vi "Update State Data.vi"(8 "error in (no error)":errorcluster, 9 "Data":variant, 10 "Argument":string, 11 "Timing Action in":refnum<class "Timing Action.lvclass">) -> (0 "error out":errorcluster, 3 "Timing Action out":refnum<class "Timing Action.lvclass">)   [LabVIEW 2020, in "MacroAssert.lvlib" / "Timing Action.lvclass"]
uses:
  Timing Action.lvclass
  Action Step/Action Step.lvclass
  Timing Action.lvclass/Timing Action.ctl
  Timing Action Type.ctl
  Time Unit.ctl
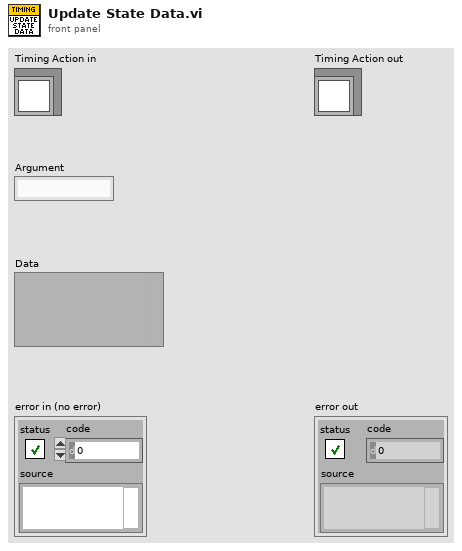
[diagram p1: front panel]
types:
  T1 = typedef "MacroAssert.lvlib/Timing Action.lvclass/Timing Action Type.ctl" = enum16{"Wait", "Wait Until"}
  T2 = typedef "MacroAssert.lvlib/Timing Action.lvclass/Time Unit.ctl" = enum16{"milliseconds", "seconds", "minutes"}
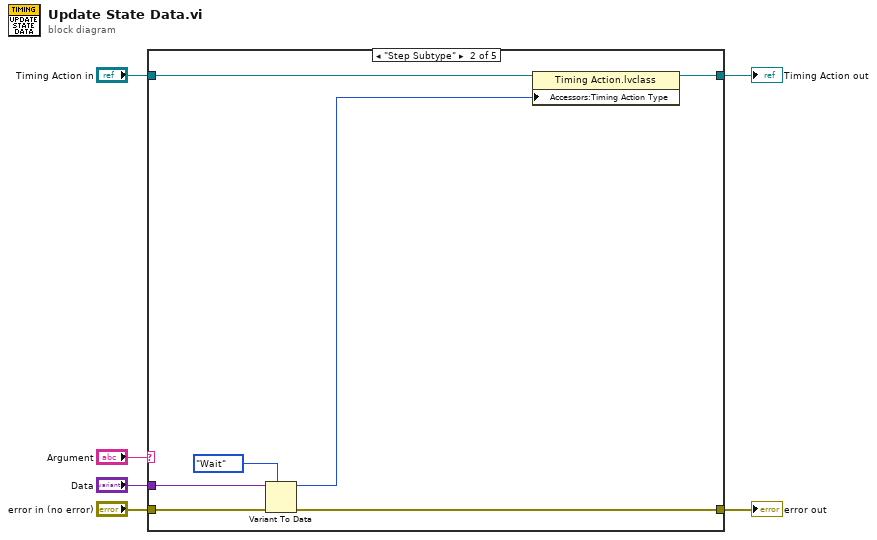
[diagram p0: block diagram]
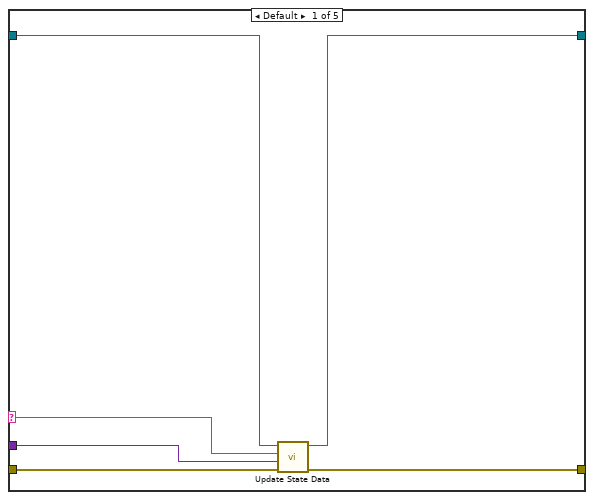
[diagram p2: hidden frame]
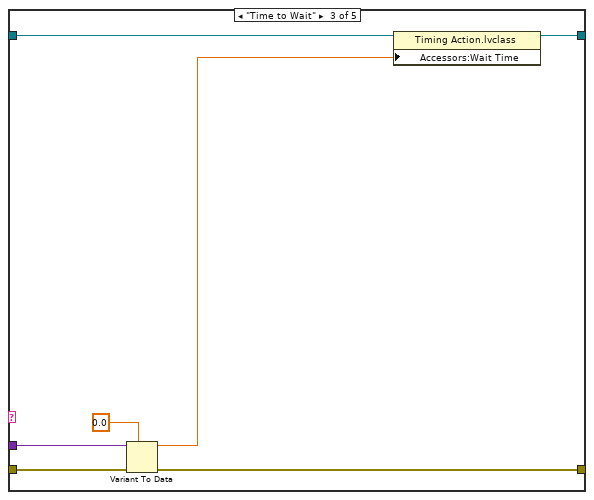
[diagram p3: hidden frame]
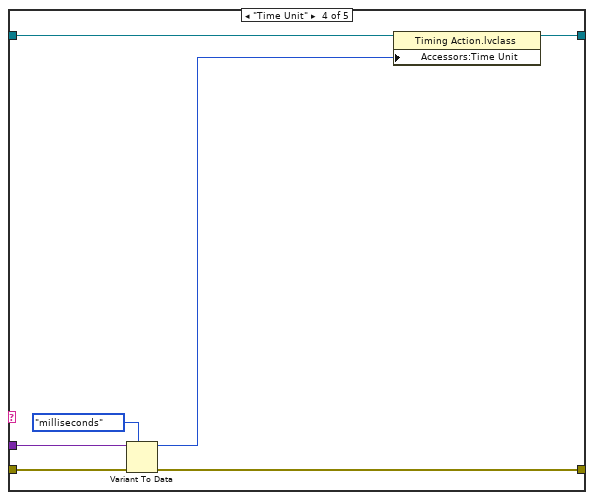
[diagram p4: hidden frame]
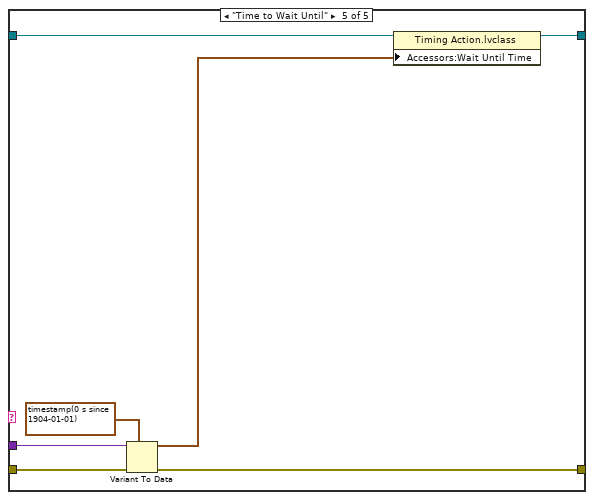
[diagram p5: hidden frame]
diagram:
  n1 = case shown="\"Step Subtype\"" "Argument" {
    selector: "Argument" -> [w9 _ _ _ _]
    tunnel: "Timing Action in" -> [w8 w19 w26 w33 w40]
    tunnel: "error in (no error)" -> [w12 w17 w24 w31 w38]
    tunnel: [w7 w18 w25 w32 w39] -> w3
    tunnel: [w11 w16 w23 w30 w37] -> w5
    tunnel: "Data" -> [w10 w14 w22 w29 w36]
    frame Default {
      n2 = call-parent "Update State Data.vi"("error in (no error)"=w12, "Data"=w10, "Argument"=w9, "Step in"=w8) -> ("error out"=w11:errorcluster, "Step out"=w7:refnum<class "Timing Action.lvclass">)  [unwired: 6 in]
    }
    frame "Step Subtype" {
      n3 = Variant To Data(error in=w17, type=Timing_Action_Type."Wait" ("Timing Action Type"), Variant=w14) -> (data=w13:T1, error out=w16:errorcluster)
      n4 = property class="Timing Action.lvclass"(reference=w19, "Accessors:Timing Action Type"=w13) -> (reference out=w18:refnum<class "Timing Action.lvclass">)  [unwired: 1 in, 1 out]
    }
    frame "Time to Wait" {
      n5 = Variant To Data(error in=w24, type=0.0, Variant=w22) -> (data=w21:dbl, error out=w23:errorcluster)
      n6 = property class="Timing Action.lvclass"(reference=w26, "Accessors:Wait Time"=w21) -> (reference out=w25:refnum<class "Timing Action.lvclass">)  [unwired: 1 in, 1 out]
    }
    frame "Time Unit" {
      n7 = Variant To Data(error in=w31, type=Time_Unit."milliseconds", Variant=w29) -> (data=w28:T2, error out=w30:errorcluster)
      n8 = property class="Timing Action.lvclass"(reference=w33, "Accessors:Time Unit"=w28) -> (reference out=w32:refnum<class "Timing Action.lvclass">)  [unwired: 1 in, 1 out]
    }
    frame "Time to Wait Until" {
      n9 = Variant To Data(error in=w38, type=timestamp(0 s since 1904-01-01), Variant=w36) -> (data=w35:timestamp, error out=w37:errorcluster)
      n10 = property class="Timing Action.lvclass"(reference=w40, "Accessors:Wait Until Time"=w35) -> (reference out=w39:refnum<class "Timing Action.lvclass">)  [unwired: 1 in, 1 out]
    }
  }
  "error out" <- w5
  "Timing Action out" <- w3
